vi "span_center_from_min_max.vi"(3 "No Points":i32, 4 "Begin":dbl, 5 "End":dbl) -> (0 "Step":dbl, 1 "Mid Point":dbl, 2 "Difference (abs)":dbl)   [LabVIEW 2013]
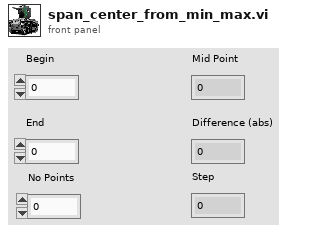
[diagram p1: front panel]
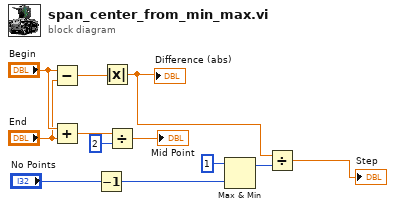
[diagram p0: block diagram]
diagram:
  n1 = Subtract(x="Begin", y="End") -> (x-y=w7:dbl)
  n2 = Add(x="Begin", y="End") -> (x+y=w9:dbl)
  n3 = Decrement(x="No Points") -> (x-1=w5:i32)
  n4 = Absolute Value(x=w7) -> (abs(x)=w2:dbl)
  "Difference (abs)" <- w2
  n5 = Divide(x=w9, y=2) -> (x/y=→"Mid Point":dbl)
  n6 = Max & Min(x=1, y=w5) -> (max(x,y)=w3:i32)  [unwired: 1 out]
  n7 = Divide(x=w2, y=w3) -> (x/y=→"Step":dbl)
